vi "配置读取.vi"(8 "error in (no error)":errorcluster) -> (0 "error out":errorcluster)   [LabVIEW 2022 SP3, in "斯坦道CODMn.lvlib"]
uses:
  <vilib>/Utility/config.llb/NI_LVConfig.lvlib
  <userlib>/_OpenG.lib/variantconfig/variantconfig.llb/openg_variant_configuration_file.lvlib
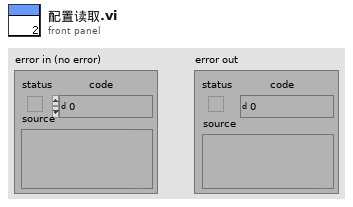
[diagram p1: front panel]
types:
  T1 = typedef "NI_LVConfig.lvlib/Config Data RefNum.ctl" = refnum<k1>
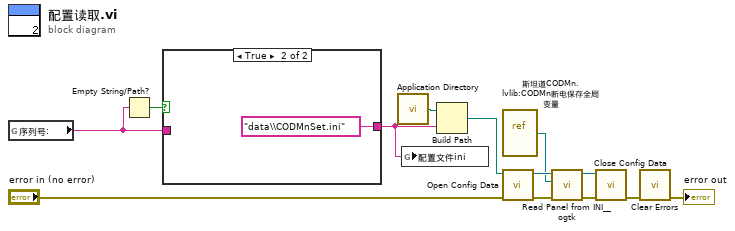
[diagram p0: block diagram]
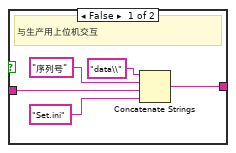
[diagram p2: hidden frame]
diagram:
  n1 = global read "COD内部交互全局.vi" "序列号:"() -> (w3:string)
  n2 = Empty String/Path?(string/path=w3) -> (empty?=w12:bool)
  n3 = case shown="True" w12 {
    tunnel: w3 -> [w15 _]
    tunnel: [w14 "data\\CODMnSet.ini" ("名称或相对路径")] -> w9
    frame False {
      # "与生产用上位机交互"
      n4 = Concatenate Strings("data\\" ("字符串"), "序列号" ("字符串"), w15, "Set.ini" ("名称或相对路径")) -> (w14:string)
    }
    frame True {
    }
  }
  n5 = call <vilib>:"Application Directory.vi"() -> ("Application Directory"=w13:path)
  n6 = global write "COD内部交互全局.vi" "配置文件ini"(w9) -> ()
  n7 = Build Path(base path=w13, name or relative path=w9) -> (appended path=w10:path)
  n8 = vi-ref "斯坦道CODMn.lvlib:CODMn断电保存全局变量.vi"() -> (w4:refnum<vi>)
  n9 = call <vilib>:"Open Config Data.vi"("error in (no error)"="error in (no error)", "configuration file path"=w10) -> ("error out"=w8:errorcluster, "refnum"=w7:T1)  [unwired: 7 in, 1 out]
  n10 = call <userlib>:"Read Panel from INI__ogtk.vi"("error in (no error)"=w8, "VI ref"=w4, "refnum"=w7) -> ("error out"=w6:errorcluster, "refnum out"=w5:T1)  [unwired: 7 in]
  n11 = call <vilib>:"Close Config Data.vi"("error in (no error)"=w6, "refnum"=w5) -> ("error out"=w11:errorcluster)  [unwired: 8 in, 1 out]
  n12 = call <vilib>:"Clear Errors.vi"("error in (no error)"=w11) -> ("error out"=→"error out":errorcluster)  [unwired: 5 in, 1 out]
